vi "Filter.vi"(1 "Bits":i16[](array[numeric]), 2 "Oversampling Factor":i32, 3 "Vref":dbl) -> (0 "Sample":dbl)   [LabVIEW 2014]
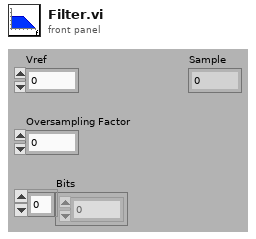
[diagram p1: front panel]
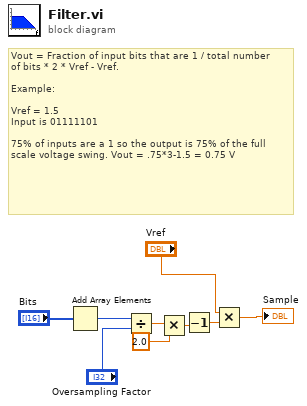
[diagram p0: block diagram]
diagram:
  # "Vout = Fraction of input bits that are 1 / total number\nof bits * 2 * Vref - Vref.\n\nExample:\n\nVref = 1.5\nInput is 01111101\n\n75% of inputs are a 1 so the output is 75% of the full\nscale voltage swing. Vout = .75*3-1.5 = 0.75 V"
  n1 = Add Array Elements(numeric array="Bits") -> (sum=w4:i16)
  n2 = Divide(x=w4, y="Oversampling Factor") -> (x/y=w3:dbl)
  n3 = Multiply(x=w3, y=2.0) -> (x*y=w2:dbl)
  n4 = Decrement(x=w2) -> (x-1=w9:dbl)
  n5 = Multiply(x="Vref", y=w9) -> (x*y=→"Sample":dbl)
